vi "PH_PILS.PC _TristateNormal.vi"(0 "i ref in":refnum<vi>, 2 "serviceName":string, 3 "Value":i32, 5 "error IO":errorcluster) -> (14 "i ref out":refnum<vi>, 19 "error out":errorcluster)   [LabVIEW 2014, in "PH_PILS.lvlib"]
uses:
  PH_PILS.lvlib
  PH_Common/PH_Common.lvlib
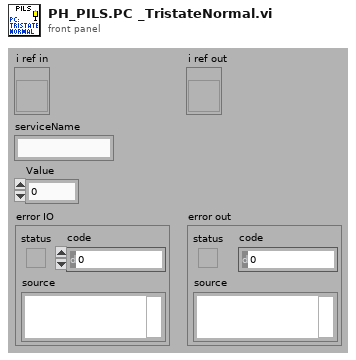
[diagram p1: front panel]
types:
  T1 = typedef "PH_PILS.lvlib/PH_PILS.i attribute.ctl" = cluster{"Boolean":cluster{"GUI Ref":refnum<vi>, "Status":i32}[], "GUI Refs Exp. Shutters":cluster{"1":refnum<vi>, "2":refnum<vi>, "3":refnum<vi>, "4":refnum<vi>}, "Tristate2Run GUI Refs":refnum<vi>[], "EO-Likes":cluster{"GUI Ref":refnum<vi>, "Status":i32}[], "Operation Mode":cluster{"Operation Mode":T2, "GUI":cluster{"Ref State":refnum<vi>, "Ref":refnum<vi>}, "Servicemode":cluster{"Tagname":string, "Status":i32}, "Labormode":cluster{"Tagname":string, "Status":i32}, "Searchmode":cluster{"Tagname":string, "Status":i32}, "Shotmode":cluster{"Tagname":string, "Status":i32}}, "Submode":cluster{"Submode":T3, "GUI":cluster{"Ref State":refnum<vi>, "Ref":refnum<vi>}, "Submode":cluster{"Tagname":string, "Status":i32}}, "Experiment":cluster{"Experiment":enum16{"unknown", "intern", "4 (Z6)", "3", "2", "1"}, "GUI":cluster{"Ref State":refnum<vi>, "Ref":refnum<vi>}, "intern":cluster{"Tagname":string, "Status":i32}, "Exp 4":cluster{"Tagname":string, "Status":i32}, "Exp 3":cluster{"Tagname":string, "Status":i32}, "Exp 2":cluster{"Tagname":string, "Status":i32}, "Exp 1":cluster{"Tagname":string, "Status":i32}}, "TristateNormal":cluster{"GUI Ref":refnum<vi>, "Status":i32}[], "Door Tags":cluster{"GUI Ref":refnum<vi>, "Status":i32}[], "GUIlessTags":cluster{"Name":string, "Status":i32}[], "Beamline GUI Refs":refnum<vi>[], "Special Boolean":cluster{"GUI Ref":refnum<vi>, "Status":i32}[], "Laserpower":cluster{"GUI Ref":refnum<vi>, "Status":i32}[], "Shutter":cluster{"GUI Ref":refnum<vi>, "Status":i32}[], "Tristate EO Like":cluster{"GUI Ref":refnum<vi>, "Status":i32}[], "PP":cluster{"GUI Ref":refnum<vi>, "Status":i32, "Head Ref":refnum<vi>, "Slider Ref":refnum<vi>}[], "Switch Knobs":cluster{"GUI Ref":refnum<vi>, "Status":i32}[], "Latch Knob GUI Refs":refnum<vi>[], "FailureCounter":i32, "Enabled Status":cluster{"Laser":i32, "PreAmp":i32, "MainAmp":i32}, "Mercury":refnum<vi>, "Instance Rods":string, "Logfile":path, "Beckhoff-Instance Internal":string, "Beckhoff-Instance External":string, "Enabling Rights":cluster{"Name":string, "Password":string, "PA?":bool, "MA?":bool, "Exp?":bool}[]}
  T2 = typedef "PH_PILS.lvlib/PH_PILS.Operation Mode.ctl" = enum16{"unknown", "Service", "Labor", "Search", "Shot"}
  T3 = typedef "PH_PILS.lvlib/PH_PILS.Submode.ctl" = enum16{"unknown", "HV-Normal", "HV-Test"}
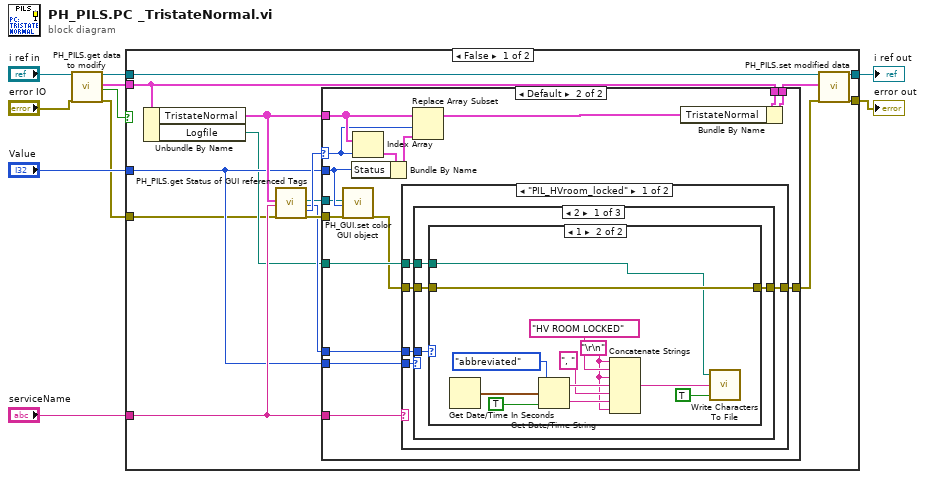
[diagram p0: block diagram]
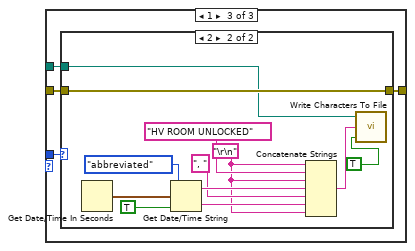
[diagram p5: hidden frame]
diagram:
  n1 = call "PH_PILS.get data to modify.vi"("i ref in"="i ref in", "error in (no error)"="error IO") -> ("i ref out"=w4:refnum<vi>, "i attribute"=w5:T1, "timed out"=w1:bool, "error out"=w6:errorcluster)  [unwired: 14 in]
  n2 = case shown="False" w1 {
    tunnel: "Value" -> [w15 _]
    tunnel: "serviceName" -> [w17 _]
    tunnel: w6 -> [w12 w85]
    tunnel: w5 -> [w14 _]
    tunnel: w4 -> [w11 w86]
    tunnel: [w25 w86] -> w3
    tunnel: [w23 w85] -> w2
    frame False {
      n3 = Unbundle By Name(w14) -> ("TristateNormal"=w21:cluster{"GUI Ref":refnum<vi>, "Status":i32}[], "Logfile"=w13:path)
      n4 = call "PH_PILS.get Status of GUI referenced Tags.vi"("Tags"=w21, "Tagname"=w17, "error in"=w12) -> ("GUI Ref"=w18:refnum<vi>, "Status"=w16:i32, "index of element"=w20:i32, "error out"=w19:errorcluster)  [unwired: 13 in]
      n5 = case shown="Default" w20 {
        selector: w20 -> [_ w35]
        tunnel: w19 -> [w26 w43]
        tunnel: [w26 w28] -> w24
        tunnel: w21 -> [_ w42]
        tunnel: w14 -> [w27 w41]
        tunnel: [w27 w40] -> w22
        tunnel: w15 -> [_ w36]
        tunnel: w18 -> [_ w34]
        tunnel: w17 -> [_ w33]
        tunnel: w16 -> [_ w32]
        tunnel: w15 -> [_ w31]
        tunnel: w13 -> [_ w30]
        frame -1 {
        }
        frame Default {
          n6 = call "PH_GUI.set color GUI object.vi"("GUI object Ref"=w34, "State"=w36, "error in (no error)"=w43) -> ("error out"=w29:errorcluster)  [unwired: 16 in]
          n7 = Index Array(array=w42, index=w35) -> (element=w38:cluster{"GUI Ref":refnum<vi>, "Status":i32})
          n8 = Bundle By Name(cluster=w38, "Status"=w36) -> (w37:cluster{"GUI Ref":refnum<vi>, "Status":i32})
          n9 = case shown="\"PIL_HVroom_locked\"" w33 {
            tunnel: w32 -> [w47 _]
            tunnel: w31 -> [w48 _]
            tunnel: w30 -> [w46 _]
            tunnel: w29 -> [w45 w84]
            tunnel: [w44 w84] -> w28
            frame "PIL_HVroom_locked" {
              n10 = case shown="2" w48 {
                tunnel: w47 -> [w52 _ w70]
                tunnel: w46 -> [w51 _ w69]
                tunnel: w45 -> [w49 w66 w68]
                tunnel: [w50 w66 w67] -> w44
                frame 2 {
                  n11 = case shown="1" w52 {
                    tunnel: w51 -> [_ w55]
                    tunnel: [w53 w56] -> w50
                    tunnel: w49 -> [w53 w56]
                    frame Default {
                    }
                    frame 1 {
                      w58 = "\r\n"
                      n12 = Get Date/Time In Seconds() -> (seconds since 1Jan1904=w64:timestamp)
                      n13 = Get Date/Time String(date format (0)=enum16{"short", "long", "abbreviated"}."abbreviated", seconds (now)=w64, want seconds? (F)=TRUE) -> (date string=w62:string, time string=w61:string)
                      n14 = Concatenate Strings(w58, "HV ROOM LOCKED" ("string"), w58, w62, ", ", w61, w58) -> (w57:string)
                      n15 = call <vilib>:"Write Characters To File.vi"("append to file? (new file:F)"=TRUE, "character string"=w57, "file path (dialog if empty)"=w55) -> ()  [unwired: 2 in, 1 out]
                    }
                  }
                }
                frame Default {
                }
                frame 1 {
                  n16 = case shown="2" w70 {
                    tunnel: w69 -> [_ w74]
                    tunnel: w68 -> [w71 w75]
                    tunnel: [w71 w75] -> w67
                    frame Default {
                    }
                    frame 2 {
                      w76 = "\r\n"
                      n17 = Get Date/Time In Seconds() -> (seconds since 1Jan1904=w82:timestamp)
                      n18 = Get Date/Time String(date format (0)=enum16{"short", "long", "abbreviated"}."abbreviated", seconds (now)=w82, want seconds? (F)=TRUE) -> (date string=w80:string, time string=w79:string)
                      n19 = Concatenate Strings(w76, "HV ROOM UNLOCKED" ("string"), w76, w80, ", ", w79, w76) -> (w73:string)
                      n20 = call <vilib>:"Write Characters To File.vi"("append to file? (new file:F)"=TRUE, "character string"=w73, "file path (dialog if empty)"=w74) -> ()  [unwired: 2 in, 1 out]
                    }
                  }
                }
              }
            }
            frame Default {
            }
          }
          n21 = Replace Array Subset(array=w42, new element=w37, index=w35) -> (w39:cluster{"GUI Ref":refnum<vi>, "Status":i32}[])
          n22 = Bundle By Name(cluster=w41, "TristateNormal"=w39) -> (w40:T1)
        }
      }
      n23 = call "PH_PILS.set modified data.vi"("i ref in"=w11, "i attribute"=w22, "error in (no error)"=w24) -> ("i ref out"=w25:refnum<vi>, "error out"=w23:errorcluster)  [unwired: 15 in]
    }
    frame True {
    }
  }
  "error out" <- w2
  "i ref out" <- w3
